vi "NanotecSMCPDDriver.find reference.vi"(0 "VISA resource name":refnum<visa-resource-name>, 1 "contollerID":i32=-1, 3 "forwardSwitch":bool, 5 "error in (no error)":errorcluster) -> (14 "VISA resource name out":refnum<visa-resource-name>, 15 "contollerID out":i32=-1, 19 "error out":errorcluster)   [LabVIEW 2014, in "NanotecSMCPDDriver.lvlib"]
doc: "Performs a movement to the reference position at the backward or forward limit switch. When using this VI, the controller should be in state \"ready\". This VI just starts the movement. It does not wait until the reference move has finished."
uses:
  NanotecSMCPDDriver.lvlib
  Private/NanotecSMCPDDriver.positioning mode types.ctl
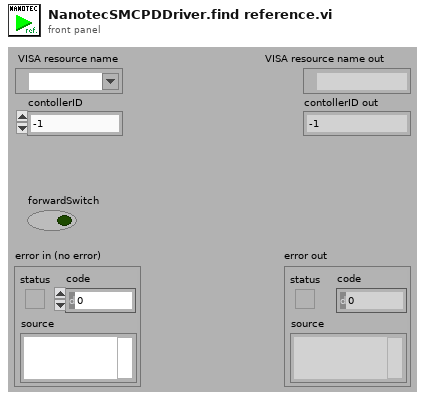
[diagram p1: front panel]
types:
  T1 = typedef "NanotecSMCPDDriver.lvlib/NanotecSMCPDDriver.positioning mode types.ctl" = enum16{"unknown", "relative positioning", "absolute positioning", "internal referencing", "external referencing"}
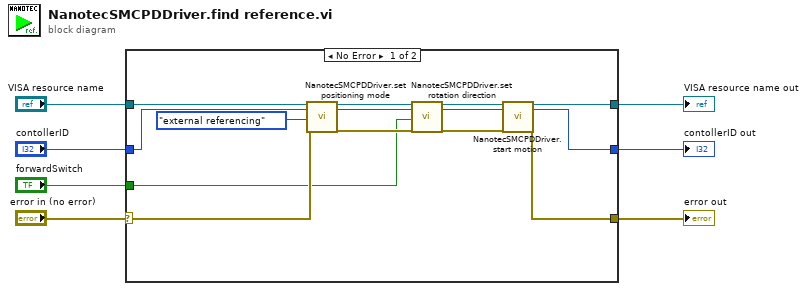
[diagram p0: block diagram]
diagram:
  n1 = case shown="No Error" "error in (no error)" {
    selector: "error in (no error)" -> [w16 w22]
    tunnel: [w20 w24] -> w7
    tunnel: [w17 w22] -> w6
    tunnel: "VISA resource name" -> [w21 w24]
    tunnel: "contollerID" -> [w19 w23]
    tunnel: [w18 w23] -> w3
    tunnel: "forwardSwitch" -> [w8 _]
    frame No Error {
      n2 = call "NanotecSMCPDDriver.set positioning mode.vi"("VISA resource name"=w21, "contollerID"=w19, "positioningMode"=NanotecSMCPDDriver.positioning_mode_types."external referencing", "error in (no error)"=w16) -> ("VISA resource name out"=w14:refnum<visa-resource-name>, "contollerID out"=w11:i32, "error out"=w10:errorcluster)  [unwired: 13 in]
      n3 = call "NanotecSMCPDDriver.set rotation direction.vi"("VISA resource name"=w14, "contollerID"=w11, "clock-wise"=w8, "error in (no error)"=w10) -> ("VISA resource name out"=w13:refnum<visa-resource-name>, "contollerID out"=w12:i32, "error out"=w9:errorcluster)  [unwired: 13 in]
      n4 = call "NanotecSMCPDDriver.start motion.vi"("VISA resource name"=w13, "contollerID"=w12, "error in (no error)"=w9) -> ("VISA resource name out"=w20:refnum<visa-resource-name>, "contollerID out"=w18:i32, "error out"=w17:errorcluster)  [unwired: 14 in]
    }
    frame Error {
    }
  }
  "VISA resource name out" <- w7
  "error out" <- w6
  "contollerID out" <- w3
